vi "Resideo Parse Data.vi"(8 "error in (no error)":errorcluster, 10 "LDO Data":u16[](array[numeric]), 11 "Vesta Data 1":u16[](array[numeric])) -> (0 "error out":errorcluster, 2 "Vesta Is Working":bool, 3 "Vesta Data Output":T1)   [LabVIEW 2020]
uses:
  Type Definitions/Vesta Info.ctl
panel:
  in  "Vesta Data":T1
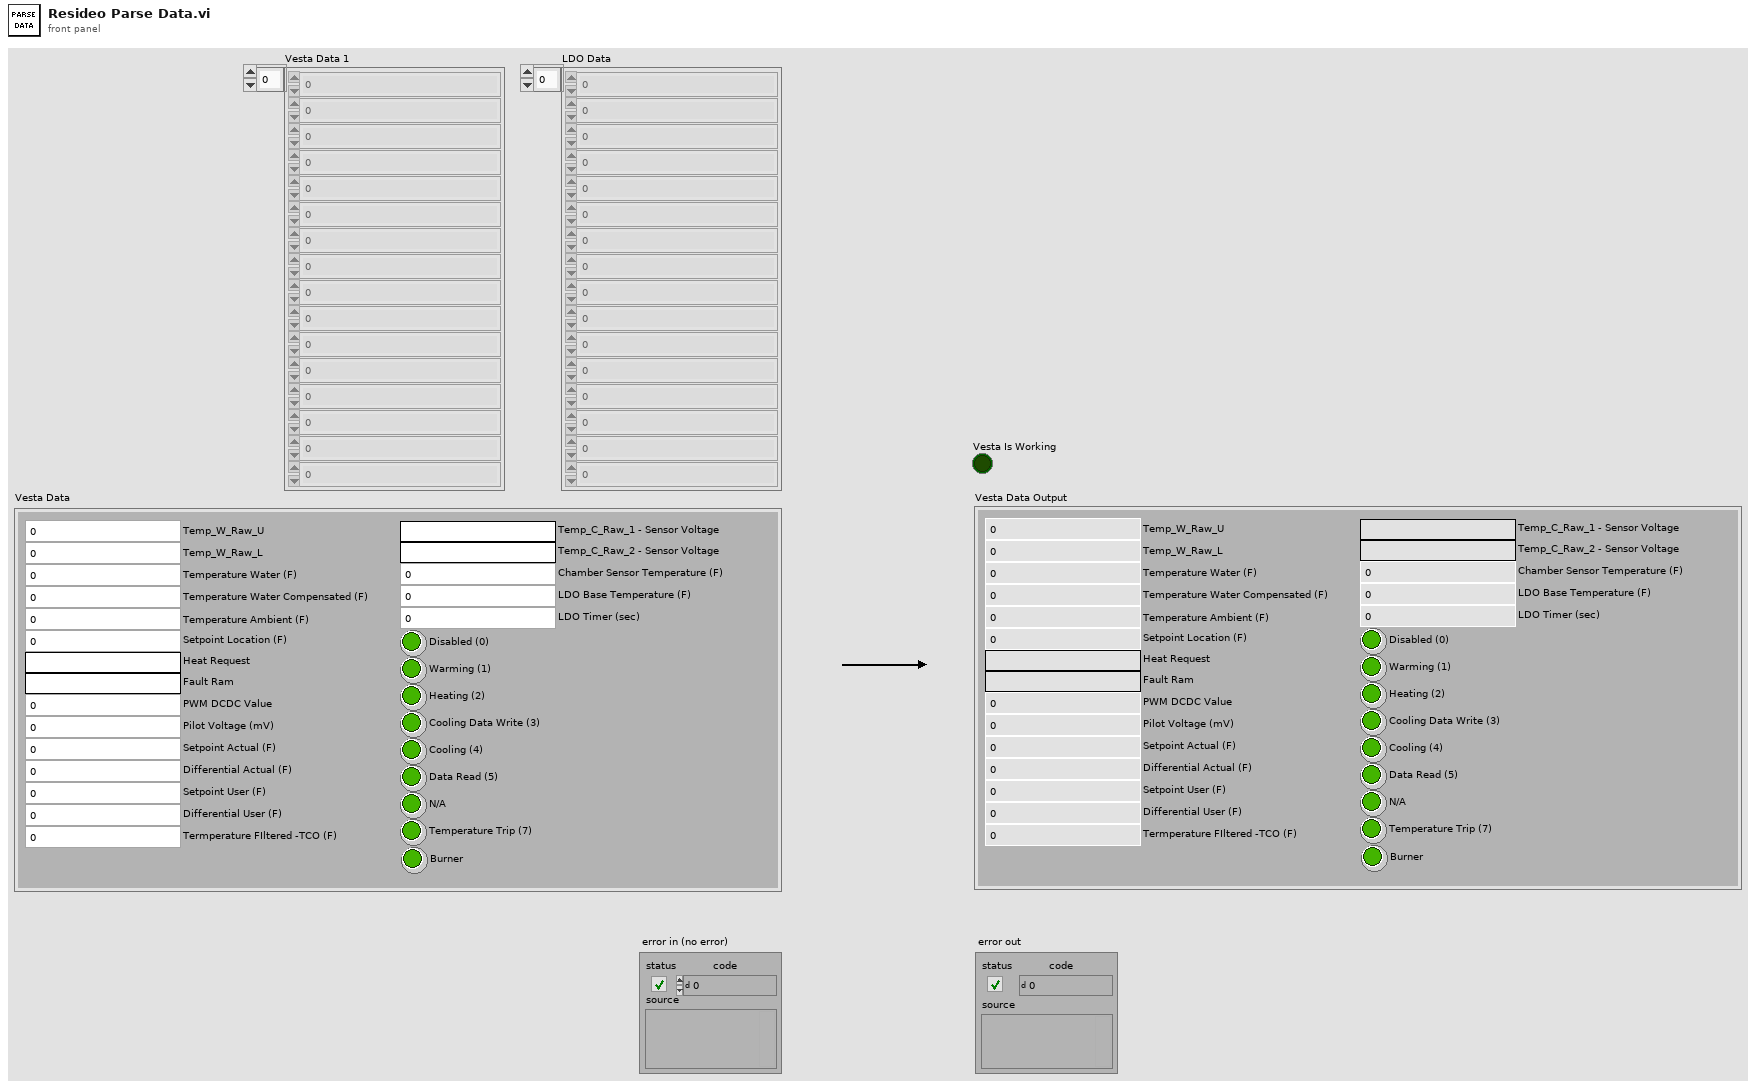
[diagram p1: front panel]
types:
  T1 = typedef "Vesta Info.ctl" = cluster{"Temp_W_Raw_U":u16, "Temp_W_Raw_L":u16, "Temperature Water (F)":dbl, "Temperature Water Compensated (F)":dbl, "Temperature Ambient (F)":dbl, "Setpoint Location (F)":dbl, "Heat Request":string, "Fault Ram":string, "PWM DCDC Value":u16, "Pilot Voltage (mV)":dbl, "Setpoint Actual (F)":dbl, "Differential Actual (F)":dbl, "Setpoint User (F)":dbl, "Differential User (F)":dbl, "Termperature FIltered -TCO (F)":dbl, "Temp_C_Raw_1 - Sensor Voltage":string, "Temp_C_Raw_2 - Sensor Voltage":string, "Chamber Sensor Temperature (F)":dbl, "LDO Base Temperature (F)":dbl, "LDO Timer (sec)":i16, "Disabled (0)":bool, "Warming (1)":bool, "Heating (2)":bool, "Cooling Data Write (3)":bool, "Cooling (4)":bool, "Data Read (5)":bool, "N/A":bool, "Temperature Trip (7)":bool, "Burner":bool}
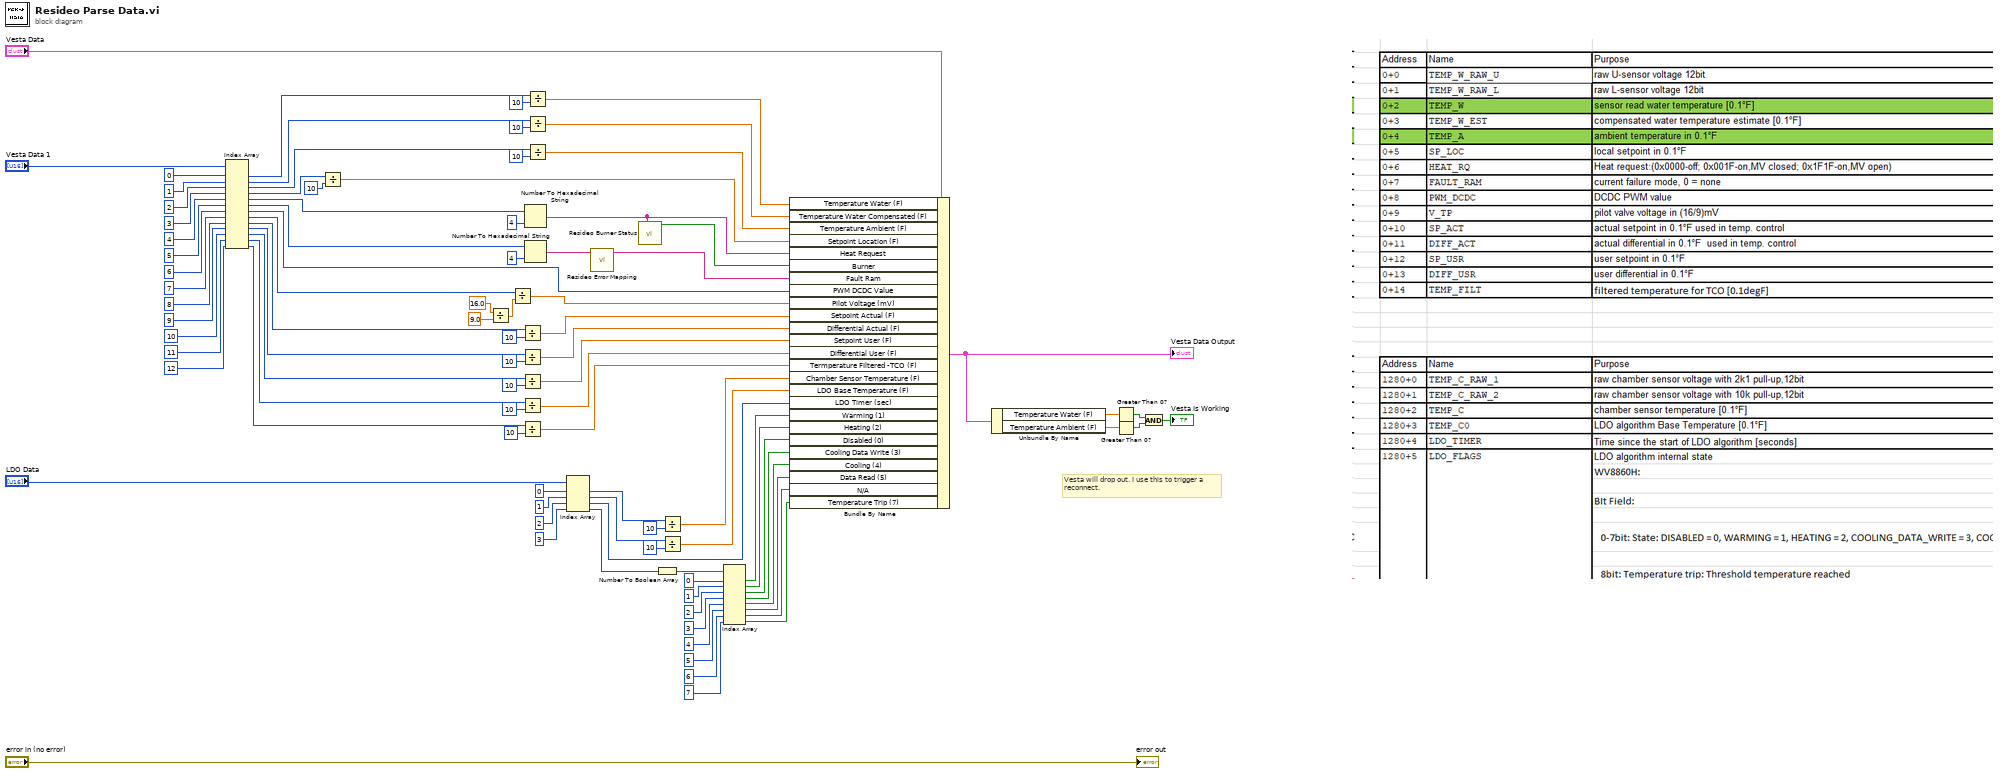
[diagram p0: block diagram]
diagram:
  # "Vesta will drop out. I use this to trigger a \nreconnect."
  n1 = Index Array(array="Vesta Data 1", index #1=0 ("index"), index #2=1 ("index"), index #3=2 ("index"), index #4=3 ("index"), index #5=4 ("index"), index #6=5 ("index"), index #7=6 ("index"), index #8=7 ("index"), index #9=8 ("index"), index #10=9 ("index"), index #11=10 ("index"), index #12=11 ("index"), index #13=12 ("index")) -> (element #1=w74:u16, element #2=w73:u16, element #3=w72:u16, element #4=w71:u16, element #5=w70:u16, element #6=w69:u16, element #7=w68:u16, element #8=w67:u16, element #9=w66:u16, element #10=w65:u16, element #11=w64:u16, element #12=w63:u16, element #13=w62:u16)
  n2 = Divide(x=w71, y=u16 10) -> (x/y=w75:dbl)
  n3 = Divide(x=16.0, y=9.0) -> (x/y=w50:dbl)
  n4 = Divide(x=w67, y=w50) -> (x/y=w49:dbl)
  n5 = Divide(x=w66, y=u16 10) -> (x/y=w47:dbl)
  n6 = Divide(x=w65, y=u16 10) -> (x/y=w45:dbl)
  n7 = Divide(x=w64, y=u16 10) -> (x/y=w43:dbl)
  n8 = Divide(x=w63, y=u16 10) -> (x/y=w41:dbl)
  n9 = Divide(x=w62, y=u16 10) -> (x/y=w39:dbl)
  n10 = Number To Hexadecimal String(1:i16 4 ("width (-)"), 2:w70) -> (0:w11:string)
  n11 = Number To Hexadecimal String(1:i16 4 ("width (-)"), 2:w69) -> (0:w53:string)
  n12 = Divide(x=w74, y=u16 10) -> (x/y=w61:dbl)
  n13 = Divide(x=w73, y=u16 10) -> (x/y=w58:dbl)
  n14 = Divide(x=w72, y=u16 10) -> (x/y=w56:dbl)
  n15 = Index Array(array="LDO Data", index #1=0 ("index"), index #2=1 ("index"), index #3=2 ("index"), index #4=3 ("index")) -> (element #1=w10:u16, element #2=w9:u16, element #3=w8:u16, element #4=w7:u16)
  n16 = call "Resideo Error Mapping.vi"("Error Code Number"=w53) -> ("Error Status"=w13:string)  [unwired: 10 in]
  n17 = call "Resideo Burner Status.vi"("Heat Request"=w11) -> ("Burner"=w12:bool)  [unwired: 10 in]
  n18 = Number To Boolean Array(number=w7) -> (Boolean array=w30:bool[])
  n19 = Divide(x=w10, y=u16 10) -> (x/y=w34:dbl)
  n20 = Divide(x=w9, y=u16 10) -> (x/y=w31:dbl)
  n21 = Index Array(array=w30, index #1=0 ("index"), index #2=1 ("index"), index #3=2 ("index"), index #4=3 ("index"), index #5=4 ("index"), index #6=5 ("index"), index #7=6 ("index"), index #8=7 ("index")) -> (element #1=w21:bool, element #2=w20:bool, element #3=w19:bool, element #4=w18:bool, element #5=w17:bool, element #6=w16:bool, element #7=w15:bool, element #8=w14:bool)
  n22 = Bundle By Name(cluster="Vesta Data", "Temperature Water (F)"=w61, "Temperature Water Compensated (F)"=w58, "Temperature Ambient (F)"=w56, "Setpoint Location (F)"=w75, "Heat Request"=w11, "Burner"=w12, "Fault Ram"=w13, "PWM DCDC Value"=w68, "Pilot Voltage (mV)"=w49, "Setpoint Actual (F)"=w47, "Differential Actual (F)"=w45, "Setpoint User (F)"=w43, "Differential User (F)"=w41, "Termperature FIltered -TCO (F)"=w39, "Chamber Sensor Temperature (F)"=w34, "LDO Base Temperature (F)"=w31, "LDO Timer (sec)"=w8, "Warming (1)"=w21, "Heating (2)"=w20, "Disabled (0)"=w19, "Cooling Data Write (3)"=w18, "Cooling (4)"=w17, "Data Read (5)"=w16, "N/A"=w15, "Temperature Trip (7)"=w14) -> (w6:T1)
  "Vesta Data Output" <- w6
  n23 = Unbundle By Name(w6) -> ("Temperature Water (F)"=w5:dbl, "Temperature Ambient (F)"=w4:dbl)
  n24 = Greater Than 0?(x=w5) -> (x > 0?=w3:bool)
  n25 = Greater Than 0?(x=w4) -> (x > 0?=w2:bool)
  n26 = And(x=w3, y=w2) -> (x .and. y?=→"Vesta Is Working":bool)
  "error out" <- "error in (no error)"
